vi "Receiver HMI Main.vi"() -> ()   [LabVIEW 2025]
uses:
  <vilib>/picture/picture.llb/Draw True-Color Pixmap.vi
  <vilib>/Instr/_visa.llb/VISA Configure Serial Port (Instr).vi
panel:
  out "Wire":bool
  out "Speaker":bool
  out "Motor":bool
  out "Light":bool
  out "Touch":bool
  out "Solenoid":bool
  out "Cancelled":bool
  out "Receive Buffer":string
  in  "Enable Wire":bool
  in  "Enable Speaker":bool
  in  "Enable Motor":bool
  in  "Enable Light":bool
  in  "Enable Touch":bool
  in  "Enable Solenoid":bool
  out "String":string
  out "2D Picture":picture
  out "Receiving Progress:":dbl(slide) scale=0.0..100.0
  # "RECEIVER"
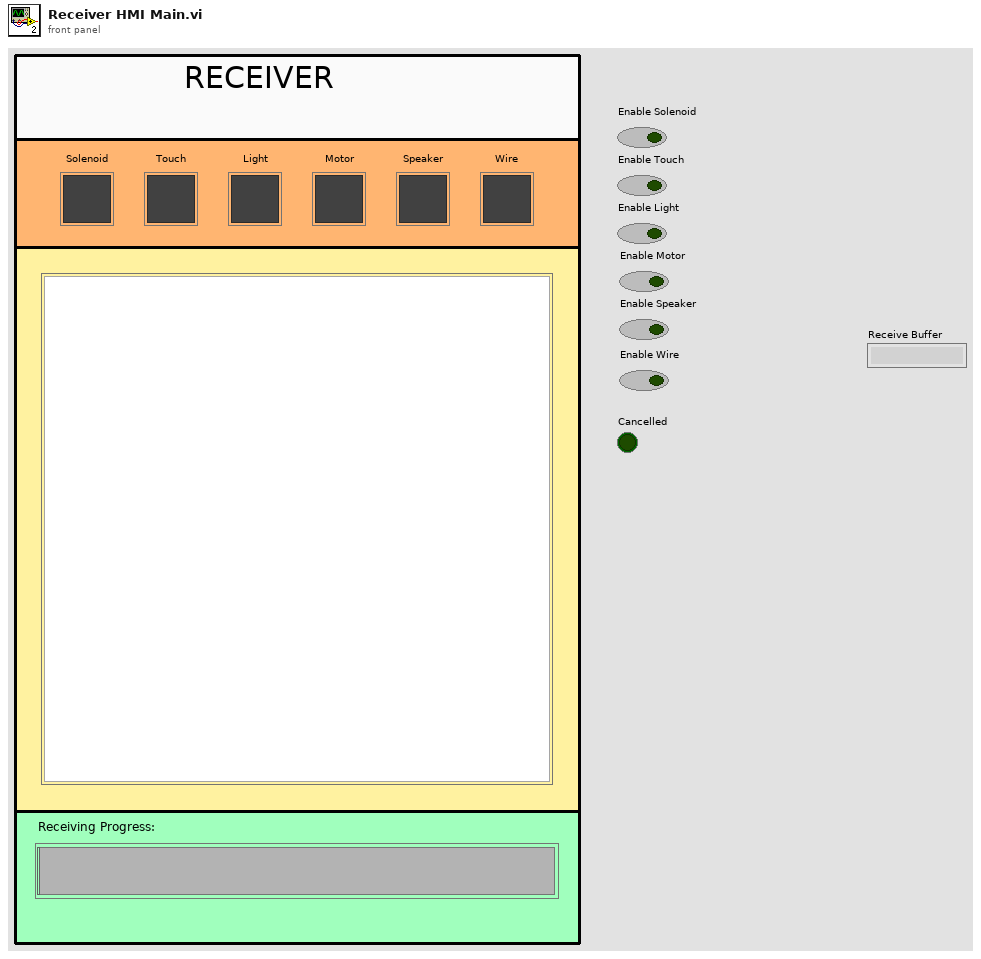
[diagram p1: front panel]
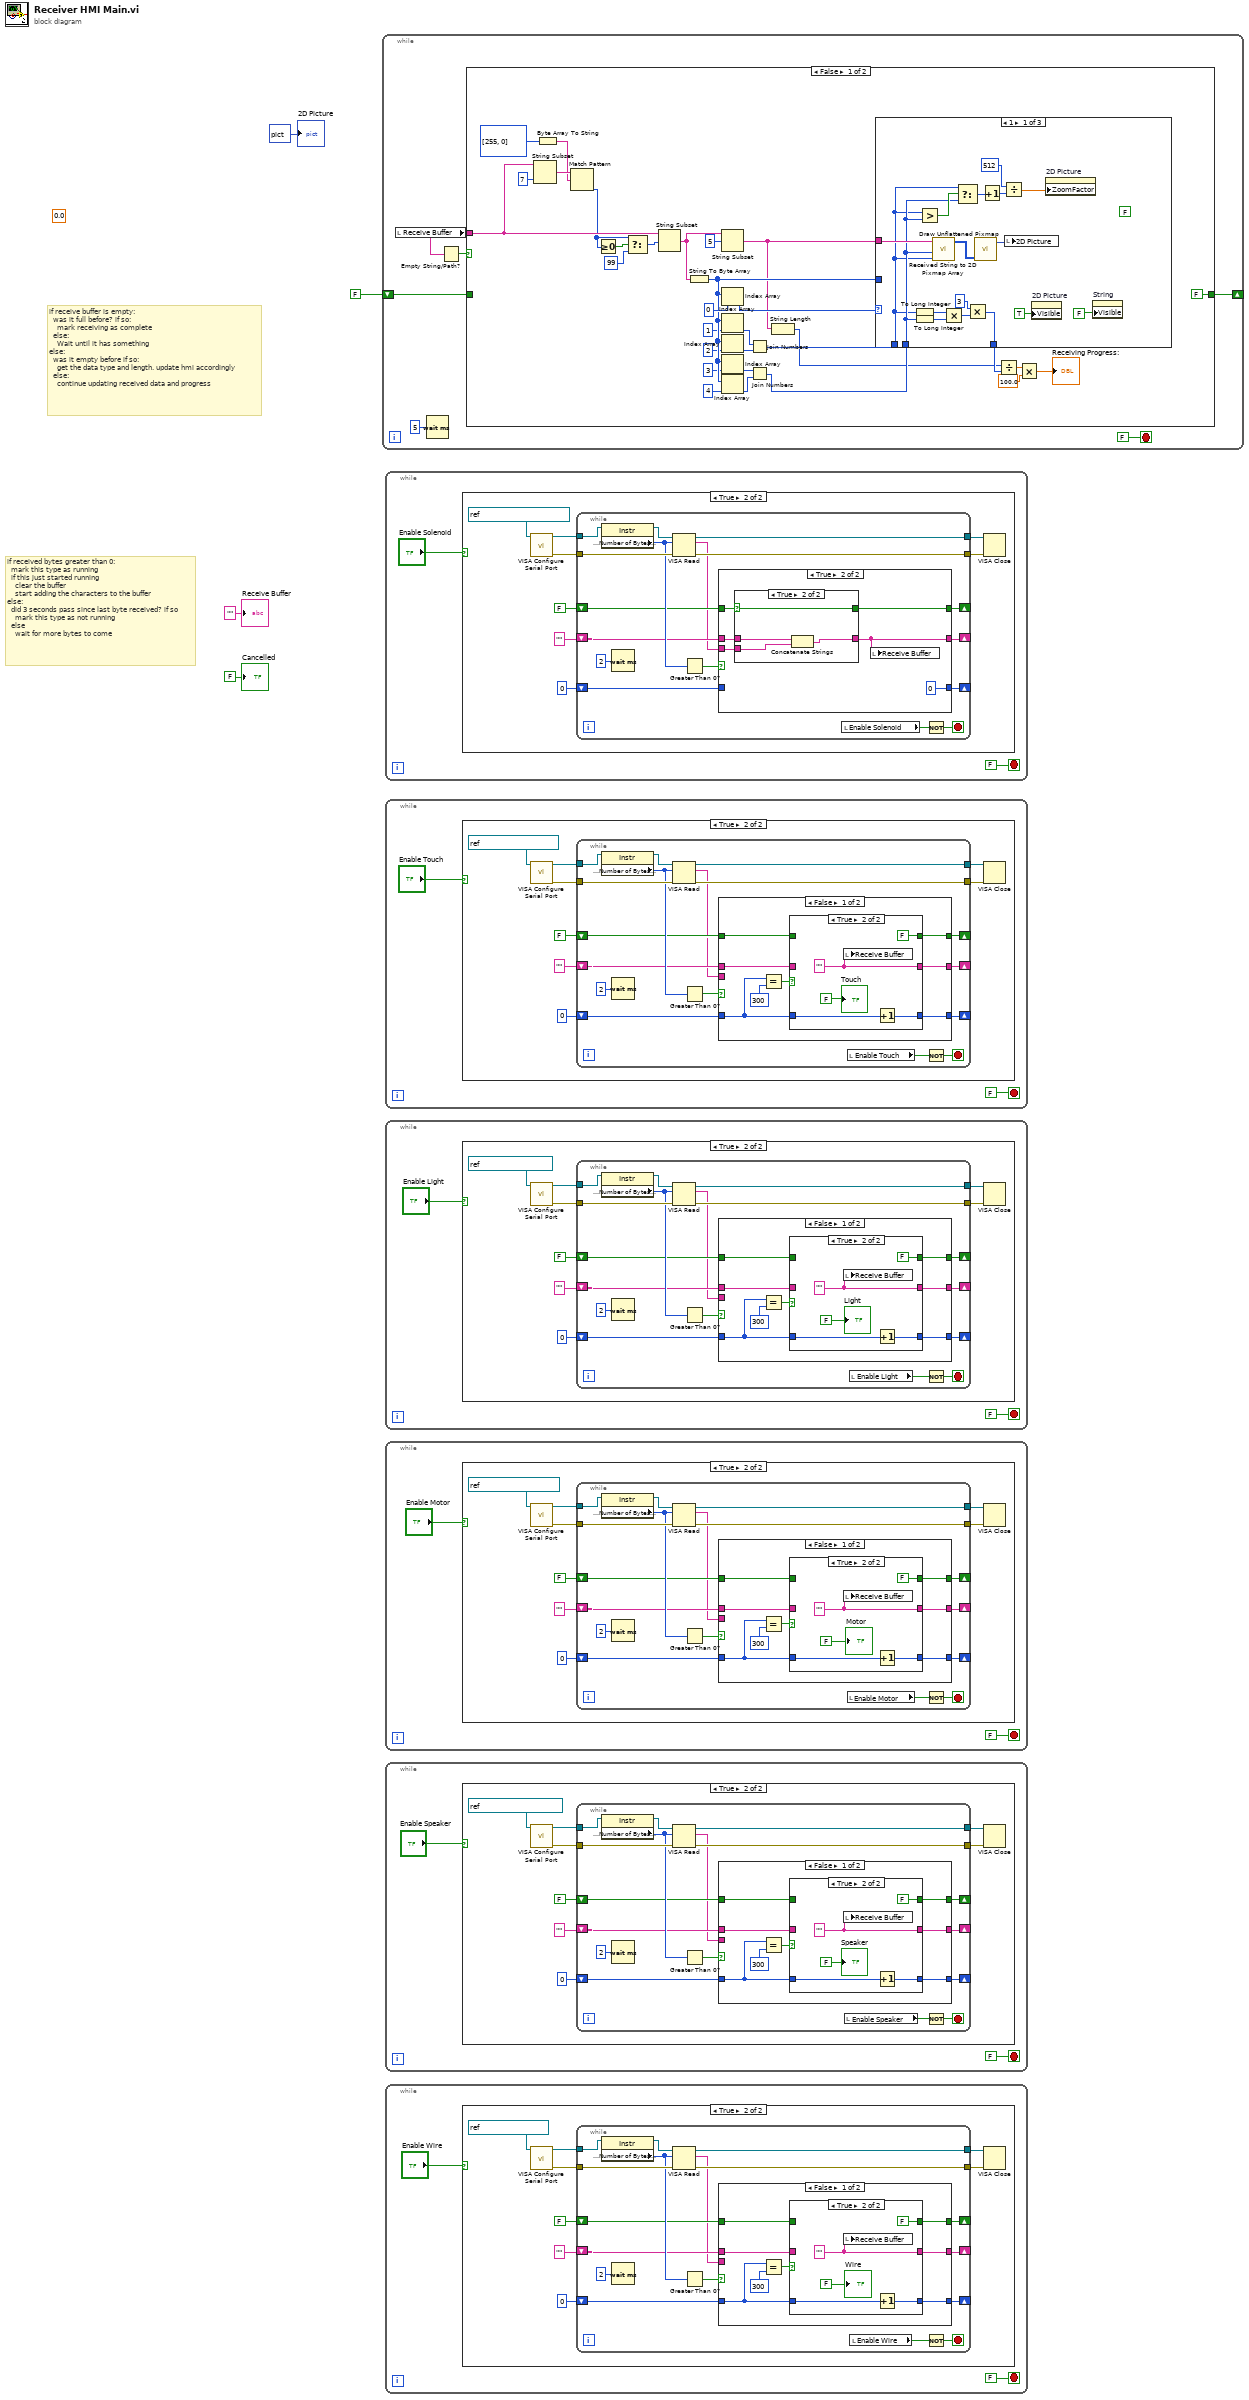
[diagram p0: block diagram]
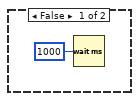
[diagram p2: hidden frame]
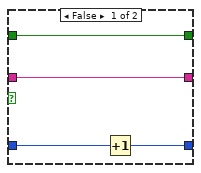
[diagram p3: hidden frame]
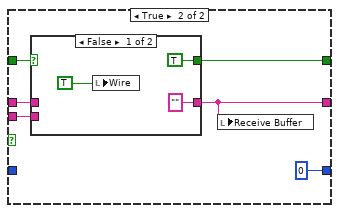
[diagram p4: hidden frame]
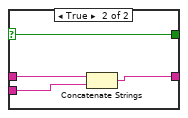
[diagram p5: hidden frame]
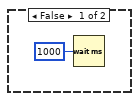
[diagram p6: hidden frame]
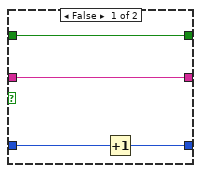
[diagram p7: hidden frame]
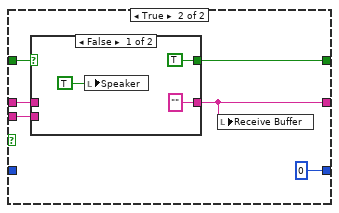
[diagram p8: hidden frame]
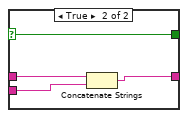
[diagram p9: hidden frame]
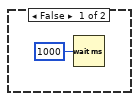
[diagram p10: hidden frame]
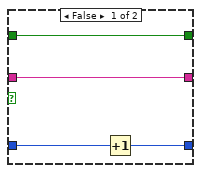
[diagram p11: hidden frame]
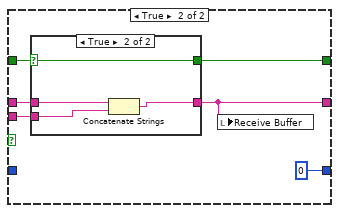
[diagram p12: hidden frame]
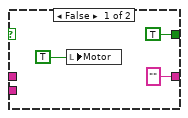
[diagram p13: hidden frame]
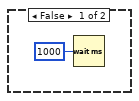
[diagram p14: hidden frame]
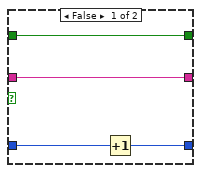
[diagram p15: hidden frame]
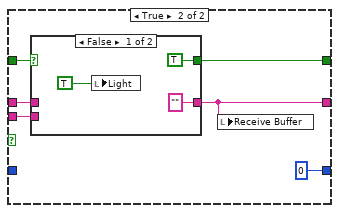
[diagram p16: hidden frame]
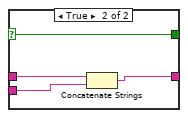
[diagram p17: hidden frame]
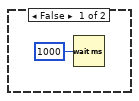
[diagram p18: hidden frame]
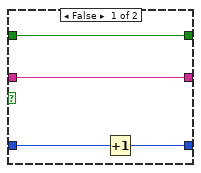
[diagram p19: hidden frame]
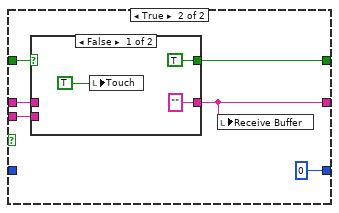
[diagram p20: hidden frame]
diagram:
  (unwired) 0.0 ("Receiving Progress:")
  # "if receive buffer is empty:\n  was it full before? if so:\n    mark receiving as complete\n  else:\n    Wait until it has something\nelse:\n  was it empty before if so:\n    get the data type and length. update hmi accordingly\n  else:\n    continue updating received data and progress"
  # "if received bytes greater than 0:\n  mark this type as running\n  if this just started running\n    clear the buffer\n    start adding the characters to the buffer\nelse:\n  did 3 seconds pass since last byte received? if so\n    mark this type as not running\n  else\n    wait for more bytes to come"
  n1 = while {
    shift-right: [w7] -> _
    shift-left: FALSE -> [w9]
    stop <- FALSE stop-if-true
    n2 = local read "Receive Buffer"() -> (w6:string)
    n3 = Wait (ms)(milliseconds to wait=u32 5) -> ()  [unwired: 1 out]
    n4 = Empty String/Path?(string/path=w6) -> (empty?=w10:bool)
    n5 = case shown="False" w10 {
      tunnel: w9 -> [_ w70]
      tunnel: [FALSE w69] -> w7
      tunnel: w6 -> [w19 _]
      frame False {
        n6 = String Subset(string=w19, length (rest)=7 ("length (rest)")) -> (substring=w21:string)  [unwired: 1 in]
        n7 = Byte Array To String(unsigned byte array=u8[] [255, 0]) -> (string=w20:string)
        n8 = Match Pattern(string=w21, regular expression=w20) -> (offset past match=w16:i32)  [unwired: 1 in, 3 out]
        n9 = Greater Or Equal To 0?(x=w16) -> (x >= 0?=w17:bool)
        n10 = Select(t=w16, s=w17, f=99) -> (s? t:f=w14:i32)
        n11 = String Subset(string=w19, offset (0)=w14) -> (substring=w18:string)  [unwired: 1 in]
        n12 = String To Byte Array(string=w18) -> (unsigned byte array=w32:u8[])
        n13 = String Subset(string=w18, offset (0)=5) -> (substring=w26:string)  [unwired: 1 in]
        n14 = Index Array(array=w32, index=0) -> (element=w40:u8)
        n15 = Index Array(array=w32, index=1) -> (element=w28:u8)
        n16 = Index Array(array=w32, index=2) -> (element=w27:u8)
        n17 = Index Array(array=w32, index=3) -> (element=w34:u8)
        n18 = Index Array(array=w32, index=4) -> (element=w33:u8)
        n19 = Join Numbers(hi=w28, lo=w27) -> ((hi.lo)=w25:u16)
        n20 = Join Numbers(hi=w34, lo=w33) -> ((hi.lo)=w24:u16)
        n21 = String Length(string=w26) -> (length=w12:i32)
        n22 = case shown="1" w40 {
          tunnel: w32 -> [_ _ _]
          tunnel: w26 -> [w56 _ w66]
          tunnel: w25 -> [w42 _ w64]
          tunnel: w24 -> [w44 _ w63]
          tunnel: [w52 u32 0 w62] -> w13
          frame 1 {
            (unwired) FALSE
            n23 = To Long Integer(number=w42) -> (32bit integer=w43:i32)
            n24 = To Long Integer(number=w44) -> (32bit integer=w45:i32)
            n25 = Greater?(x=w42, y=w44) -> (0:w50:bool)
            n26 = call "Received String to 2D Pixmap Array.vi"("Width"=w42, "Height"=w44, "Receive Buffer"=w56) -> ("Array"=w55:u32[][])  [unwired: 8 in]
            n27 = Multiply(x=w43, y=w45) -> (x*y=w54:i32)
            n28 = Select(t=w42, s=w50, f=w44) -> (s? t:f=w46:u16)
            n29 = Multiply(x=u16 3, y=w54) -> (x*y=w52:i32)
            n30 = call-poly <vilib>:"Draw Unflattened Pixmap.vi"("data (RGB format)"=w55) -> ("new picture"=w57:picture)  [unwired: 8 in]
            n31 = Increment(x=w46) -> (x+1=w47:u16)
            n32 = Divide(x=u16 512, y=w47) -> (x/y=w48:dbl)
            n33 = local write "2D Picture"(w57) -> ()
            n34 = property on="2D Picture" class="Pict"("Visible"=TRUE) -> ()  [unwired: 2 in, 2 out]
            n35 = property on="2D Picture" class="Pict"("ZoomFactor"=w48) -> ()  [unwired: 2 in, 2 out]
            n36 = property on="String" class="Str"("Visible"=FALSE) -> ()  [unwired: 2 in, 2 out]
          }
          frame Default {
            (unwired) FALSE
            n37 = local write "String"("INVALID DATA TYPE") -> ()
          }
          frame 0 {
            (unwired) TRUE
            n38 = property on="2D Picture" class="Pict"("Visible"=FALSE) -> ()  [unwired: 2 in, 2 out]
            n39 = property on="String" class="Str"("Visible"=TRUE) -> ()  [unwired: 2 in, 2 out]
            n40 = Join Numbers(hi=w64, lo=w63) -> ((hi.lo)=w62:u32)
            n41 = property on="String" class="Str"() -> ("Key Focus"=w67:bool)  [unwired: 2 in, 2 out]
            n42 = case shown="False" w67 {
              frame False {
                n43 = property on="String" class="Str"("Text.Scroll Position"=u32 65535) -> ()  [unwired: 2 in, 2 out]
              }
              frame True {
              }
            }
            "String" <- w66
          }
        }
        n44 = Divide(x=w12, y=w13) -> (x/y=w39:dbl)
        n45 = Multiply(x=w39, y=100.0) -> (x*y=→"Receiving Progress:":dbl)
      }
      frame True {
        n46 = case shown="True" w70 {
          selector: w70 -> [w71 _]
          tunnel: [w71 FALSE] -> w69
          frame False {
          }
          frame True {
            # "mark receiving as complete"
          }
        }
      }
    }
  }
  n47 = while {
    stop <- FALSE stop-if-true
    n48 = case shown="True" "Enable Solenoid" {
      frame False {
        n49 = Wait (ms)(milliseconds to wait=u32 1000) -> ()  [unwired: 1 out]
      }
      frame True {
        n50 = call-poly "VISA Configure Serial Port"("VISA resource name"=refnum<visa-resource-name> "SOLENOID_RECEIVER") -> ("VISA resource name out"=w82:refnum<visa-resource-name>, "error out"=w83:errorcluster)  [unwired: 13 in]
        n51 = while {
          tunnel: w83 -> [w100]
          tunnel: w82 -> [w98]
          shift-right: [w87] -> _
          shift-left: 0 -> [w86]
          shift-right: [w90] -> _
          shift-left: "" -> [w91]
          tunnel: [w96] -> w79
          tunnel: [w95] -> w78
          shift-right: [w88] -> _
          shift-left: FALSE -> [w92]
          stop <- w85 stop-if-true
          n52 = property class="Instr"(reference=w98) -> (reference out=w97:refnum<visa-resource-name>, "Serial Settings:Number of Bytes at Serial Port"=w93:u32)  [unwired: 1 in, 1 out]
          n53 = Wait (ms)(milliseconds to wait=u32 2) -> ()  [unwired: 1 out]
          n54 = VISA Read(VISA resource name=w97, byte count=w93, error in (no error)=w100) -> (VISA resource name out=w96:refnum<visa-resource-name>, read buffer=w89:string, error out=w95:errorcluster)  [unwired: 1 out]
          n55 = Greater Than 0?(x=w93) -> (x > 0?=w94:bool)
          n56 = case shown="True" w94 {
            tunnel: w92 -> [w101 w123]
            tunnel: w91 -> [w106 w122]
            tunnel: [w105 w118] -> w90
            tunnel: w89 -> [_ w121]
            tunnel: [w104 w120] -> w88
            tunnel: [w103 0] -> w87
            tunnel: w86 -> [w102 _]
            frame False {
              n57 = Equal?(x=w102, y=300) -> (x = y?=w107:bool)
              n58 = case shown="False" w107 {
                tunnel: w106 -> [w112 _]
                tunnel: [w112 w115] -> w105
                tunnel: [w111 FALSE] -> w104
                tunnel: [w109 w113] -> w103
                tunnel: w102 -> [w110 w114]
                tunnel: w101 -> [w111 _]
                frame False {
                  n59 = Increment(x=w110) -> (x+1=w109:i32)
                }
                frame True {
                  w115 = ""
                  n60 = local write "Receive Buffer"(w115) -> ()
                  n61 = Increment(x=w114) -> (x+1=w113:i32)
                  "Solenoid" <- FALSE ("Solenoid")
                }
              }
            }
            frame True {
              n62 = case shown="True" w123 {
                selector: w123 -> [_ w130]
                tunnel: w122 -> [_ w129]
                tunnel: ["" w128] -> w118
                tunnel: w121 -> [_ w127]
                tunnel: [TRUE w130] -> w120
                frame False {
                  n63 = local write "Solenoid"(TRUE ("Solenoid")) -> ()
                }
                frame True {
                  n64 = Concatenate Strings(w129, w127) -> (w128:string)
                }
              }
              n65 = local write "Receive Buffer"(w118) -> ()
            }
          }
          n66 = local read "Enable Solenoid"() -> (w84:bool)
          n67 = Not(x=w84) -> (.not. x?=w85:bool)
        }
        n68 = VISA Close(VISA resource name=w79, error in (no error)=w78) -> ()  [unwired: 1 out]
      }
    }
  }
  n69 = while {
    stop <- FALSE stop-if-true
    n70 = case shown="True" "Enable Touch" {
      frame False {
        n71 = Wait (ms)(milliseconds to wait=u32 1000) -> ()  [unwired: 1 out]
      }
      frame True {
        n72 = call-poly "VISA Configure Serial Port"("VISA resource name"=refnum<visa-resource-name> "TOUCH_RECEIVER") -> ("VISA resource name out"=w140:refnum<visa-resource-name>, "error out"=w141:errorcluster)  [unwired: 13 in]
        n73 = while {
          tunnel: w141 -> [w158]
          tunnel: w140 -> [w156]
          shift-right: [w145] -> _
          shift-left: 0 -> [w144]
          shift-right: [w148] -> _
          shift-left: "" -> [w149]
          tunnel: [w154] -> w137
          tunnel: [w153] -> w136
          shift-right: [w146] -> _
          shift-left: FALSE -> [w150]
          stop <- w143 stop-if-true
          n74 = property class="Instr"(reference=w156) -> (reference out=w155:refnum<visa-resource-name>, "Serial Settings:Number of Bytes at Serial Port"=w151:u32)  [unwired: 1 in, 1 out]
          n75 = Wait (ms)(milliseconds to wait=u32 2) -> ()  [unwired: 1 out]
          n76 = VISA Read(VISA resource name=w155, byte count=w151, error in (no error)=w158) -> (VISA resource name out=w154:refnum<visa-resource-name>, read buffer=w147:string, error out=w153:errorcluster)  [unwired: 1 out]
          n77 = Greater Than 0?(x=w151) -> (x > 0?=w152:bool)
          n78 = case shown="False" w152 {
            tunnel: w150 -> [w162 w181]
            tunnel: w149 -> [w166 w180]
            tunnel: [w165 w176] -> w148
            tunnel: w147 -> [_ w179]
            tunnel: [w164 w178] -> w146
            tunnel: [w163 0] -> w145
            tunnel: w144 -> [w160 _]
            frame False {
              n79 = Equal?(x=w160, y=300) -> (x = y?=w161:bool)
              n80 = case shown="True" w161 {
                tunnel: w166 -> [w170 _]
                tunnel: [w170 w174] -> w165
                tunnel: [w169 FALSE] -> w164
                tunnel: [w167 w171] -> w163
                tunnel: w160 -> [w168 w172]
                tunnel: w162 -> [w169 _]
                frame False {
                  n81 = Increment(x=w168) -> (x+1=w167:i32)
                }
                frame True {
                  w174 = ""
                  n82 = local write "Receive Buffer"(w174) -> ()
                  n83 = Increment(x=w172) -> (x+1=w171:i32)
                  "Touch" <- FALSE ("Solenoid")
                }
              }
            }
            frame True {
              n84 = case shown="False" w181 {
                selector: w181 -> [_ w188]
                tunnel: w180 -> [_ w187]
                tunnel: ["" w186] -> w176
                tunnel: w179 -> [_ w185]
                tunnel: [TRUE w188] -> w178
                frame False {
                  n85 = local write "Touch"(TRUE ("Solenoid")) -> ()
                }
                frame True {
                  n86 = Concatenate Strings(w187, w185) -> (w186:string)
                }
              }
              n87 = local write "Receive Buffer"(w176) -> ()
            }
          }
          n88 = local read "Enable Touch"() -> (w142:bool)
          n89 = Not(x=w142) -> (.not. x?=w143:bool)
        }
        n90 = VISA Close(VISA resource name=w137, error in (no error)=w136) -> ()  [unwired: 1 out]
      }
    }
  }
  n91 = while {
    stop <- FALSE stop-if-true
    n92 = case shown="True" "Enable Light" {
      frame False {
        n93 = Wait (ms)(milliseconds to wait=u32 1000) -> ()  [unwired: 1 out]
      }
      frame True {
        n94 = call-poly "VISA Configure Serial Port"("VISA resource name"=refnum<visa-resource-name> "LIGHT_RECEIVER") -> ("VISA resource name out"=w198:refnum<visa-resource-name>, "error out"=w199:errorcluster)  [unwired: 13 in]
        n95 = while {
          tunnel: w199 -> [w216]
          tunnel: w198 -> [w214]
          shift-right: [w203] -> _
          shift-left: 0 -> [w202]
          shift-right: [w206] -> _
          shift-left: "" -> [w207]
          tunnel: [w212] -> w195
          tunnel: [w211] -> w194
          shift-right: [w204] -> _
          shift-left: FALSE -> [w208]
          stop <- w201 stop-if-true
          n96 = property class="Instr"(reference=w214) -> (reference out=w213:refnum<visa-resource-name>, "Serial Settings:Number of Bytes at Serial Port"=w209:u32)  [unwired: 1 in, 1 out]
          n97 = Wait (ms)(milliseconds to wait=u32 2) -> ()  [unwired: 1 out]
          n98 = VISA Read(VISA resource name=w213, byte count=w209, error in (no error)=w216) -> (VISA resource name out=w212:refnum<visa-resource-name>, read buffer=w205:string, error out=w211:errorcluster)  [unwired: 1 out]
          n99 = Greater Than 0?(x=w209) -> (x > 0?=w210:bool)
          n100 = case shown="False" w210 {
            tunnel: w208 -> [w220 w239]
            tunnel: w207 -> [w224 w238]
            tunnel: [w223 w234] -> w206
            tunnel: w205 -> [_ w237]
            tunnel: [w222 w236] -> w204
            tunnel: [w221 0] -> w203
            tunnel: w202 -> [w218 _]
            frame False {
              n101 = Equal?(x=w218, y=300) -> (x = y?=w219:bool)
              n102 = case shown="True" w219 {
                tunnel: w224 -> [w228 _]
                tunnel: [w228 w232] -> w223
                tunnel: [w227 FALSE] -> w222
                tunnel: [w225 w230] -> w221
                tunnel: w218 -> [w226 w231]
                tunnel: w220 -> [w227 _]
                frame False {
                  n103 = Increment(x=w226) -> (x+1=w225:i32)
                }
                frame True {
                  w232 = ""
                  n104 = local write "Receive Buffer"(w232) -> ()
                  n105 = Increment(x=w231) -> (x+1=w230:i32)
                  "Light" <- FALSE ("Solenoid")
                }
              }
            }
            frame True {
              n106 = case shown="False" w239 {
                selector: w239 -> [_ w246]
                tunnel: w238 -> [_ w245]
                tunnel: ["" w244] -> w234
                tunnel: w237 -> [_ w243]
                tunnel: [TRUE w246] -> w236
                frame False {
                  n107 = local write "Light"(TRUE ("Solenoid")) -> ()
                }
                frame True {
                  n108 = Concatenate Strings(w245, w243) -> (w244:string)
                }
              }
              n109 = local write "Receive Buffer"(w234) -> ()
            }
          }
          n110 = local read "Enable Light"() -> (w200:bool)
          n111 = Not(x=w200) -> (.not. x?=w201:bool)
        }
        n112 = VISA Close(VISA resource name=w195, error in (no error)=w194) -> ()  [unwired: 1 out]
      }
    }
  }
  n113 = while {
    stop <- FALSE stop-if-true
    n114 = case shown="True" "Enable Motor" {
      frame False {
        n115 = Wait (ms)(milliseconds to wait=u32 1000) -> ()  [unwired: 1 out]
      }
      frame True {
        n116 = call-poly "VISA Configure Serial Port"("VISA resource name"=refnum<visa-resource-name> "MOTOR_RECEIVER") -> ("VISA resource name out"=w256:refnum<visa-resource-name>, "error out"=w257:errorcluster)  [unwired: 13 in]
        n117 = while {
          tunnel: w257 -> [w274]
          tunnel: w256 -> [w272]
          shift-right: [w261] -> _
          shift-left: 0 -> [w260]
          shift-right: [w264] -> _
          shift-left: "" -> [w265]
          tunnel: [w270] -> w253
          tunnel: [w269] -> w252
          shift-right: [w262] -> _
          shift-left: FALSE -> [w266]
          stop <- w259 stop-if-true
          n118 = property class="Instr"(reference=w272) -> (reference out=w271:refnum<visa-resource-name>, "Serial Settings:Number of Bytes at Serial Port"=w267:u32)  [unwired: 1 in, 1 out]
          n119 = Wait (ms)(milliseconds to wait=u32 2) -> ()  [unwired: 1 out]
          n120 = VISA Read(VISA resource name=w271, byte count=w267, error in (no error)=w274) -> (VISA resource name out=w270:refnum<visa-resource-name>, read buffer=w263:string, error out=w269:errorcluster)  [unwired: 1 out]
          n121 = Greater Than 0?(x=w267) -> (x > 0?=w268:bool)
          n122 = case shown="False" w268 {
            tunnel: w266 -> [w278 w297]
            tunnel: w265 -> [w282 w296]
            tunnel: [w281 w292] -> w264
            tunnel: w263 -> [_ w295]
            tunnel: [w280 w294] -> w262
            tunnel: [w279 0] -> w261
            tunnel: w260 -> [w276 _]
            frame False {
              n123 = Equal?(x=w276, y=300) -> (x = y?=w277:bool)
              n124 = case shown="True" w277 {
                tunnel: w282 -> [w286 _]
                tunnel: [w286 w290] -> w281
                tunnel: [w285 FALSE] -> w280
                tunnel: [w283 w288] -> w279
                tunnel: w276 -> [w284 w289]
                tunnel: w278 -> [w285 _]
                frame False {
                  n125 = Increment(x=w284) -> (x+1=w283:i32)
                }
                frame True {
                  w290 = ""
                  n126 = local write "Receive Buffer"(w290) -> ()
                  n127 = Increment(x=w289) -> (x+1=w288:i32)
                  "Motor" <- FALSE ("Solenoid")
                }
              }
            }
            frame True {
              n128 = case shown="True" w297 {
                selector: w297 -> [_ w304]
                tunnel: w296 -> [_ w303]
                tunnel: ["" w302] -> w292
                tunnel: w295 -> [_ w301]
                tunnel: [TRUE w304] -> w294
                frame False {
                  n129 = local write "Motor"(TRUE ("Solenoid")) -> ()
                }
                frame True {
                  n130 = Concatenate Strings(w303, w301) -> (w302:string)
                }
              }
              n131 = local write "Receive Buffer"(w292) -> ()
            }
          }
          n132 = local read "Enable Motor"() -> (w258:bool)
          n133 = Not(x=w258) -> (.not. x?=w259:bool)
        }
        n134 = VISA Close(VISA resource name=w253, error in (no error)=w252) -> ()  [unwired: 1 out]
      }
    }
  }
  n135 = while {
    stop <- FALSE stop-if-true
    n136 = case shown="True" "Enable Speaker" {
      frame False {
        n137 = Wait (ms)(milliseconds to wait=u32 1000) -> ()  [unwired: 1 out]
      }
      frame True {
        n138 = call-poly "VISA Configure Serial Port"("VISA resource name"=refnum<visa-resource-name> "SPEAKER_RECEIVER") -> ("VISA resource name out"=w314:refnum<visa-resource-name>, "error out"=w315:errorcluster)  [unwired: 13 in]
        n139 = while {
          tunnel: w315 -> [w332]
          tunnel: w314 -> [w330]
          shift-right: [w319] -> _
          shift-left: 0 -> [w318]
          shift-right: [w322] -> _
          shift-left: "" -> [w323]
          tunnel: [w328] -> w311
          tunnel: [w327] -> w310
          shift-right: [w320] -> _
          shift-left: FALSE -> [w324]
          stop <- w317 stop-if-true
          n140 = property class="Instr"(reference=w330) -> (reference out=w329:refnum<visa-resource-name>, "Serial Settings:Number of Bytes at Serial Port"=w325:u32)  [unwired: 1 in, 1 out]
          n141 = Wait (ms)(milliseconds to wait=u32 2) -> ()  [unwired: 1 out]
          n142 = VISA Read(VISA resource name=w329, byte count=w325, error in (no error)=w332) -> (VISA resource name out=w328:refnum<visa-resource-name>, read buffer=w321:string, error out=w327:errorcluster)  [unwired: 1 out]
          n143 = Greater Than 0?(x=w325) -> (x > 0?=w326:bool)
          n144 = case shown="False" w326 {
            tunnel: w324 -> [w336 w355]
            tunnel: w323 -> [w340 w354]
            tunnel: [w339 w350] -> w322
            tunnel: w321 -> [_ w353]
            tunnel: [w338 w352] -> w320
            tunnel: [w337 0] -> w319
            tunnel: w318 -> [w334 _]
            frame False {
              n145 = Equal?(x=w334, y=300) -> (x = y?=w335:bool)
              n146 = case shown="True" w335 {
                tunnel: w340 -> [w344 _]
                tunnel: [w344 w348] -> w339
                tunnel: [w343 FALSE] -> w338
                tunnel: [w341 w346] -> w337
                tunnel: w334 -> [w342 w347]
                tunnel: w336 -> [w343 _]
                frame False {
                  n147 = Increment(x=w342) -> (x+1=w341:i32)
                }
                frame True {
                  w348 = ""
                  n148 = local write "Receive Buffer"(w348) -> ()
                  n149 = Increment(x=w347) -> (x+1=w346:i32)
                  "Speaker" <- FALSE ("Solenoid")
                }
              }
            }
            frame True {
              n150 = case shown="False" w355 {
                selector: w355 -> [_ w362]
                tunnel: w354 -> [_ w361]
                tunnel: ["" w360] -> w350
                tunnel: w353 -> [_ w359]
                tunnel: [TRUE w362] -> w352
                frame False {
                  n151 = local write "Speaker"(TRUE ("Solenoid")) -> ()
                }
                frame True {
                  n152 = Concatenate Strings(w361, w359) -> (w360:string)
                }
              }
              n153 = local write "Receive Buffer"(w350) -> ()
            }
          }
          n154 = local read "Enable Speaker"() -> (w316:bool)
          n155 = Not(x=w316) -> (.not. x?=w317:bool)
        }
        n156 = VISA Close(VISA resource name=w311, error in (no error)=w310) -> ()  [unwired: 1 out]
      }
    }
  }
  n157 = while {
    stop <- FALSE stop-if-true
    n158 = case shown="True" "Enable Wire" {
      frame False {
        n159 = Wait (ms)(milliseconds to wait=u32 1000) -> ()  [unwired: 1 out]
      }
      frame True {
        n160 = call-poly "VISA Configure Serial Port"("VISA resource name"=refnum<visa-resource-name> "WIRE_RECEIVER") -> ("VISA resource name out"=w372:refnum<visa-resource-name>, "error out"=w373:errorcluster)  [unwired: 13 in]
        n161 = while {
          tunnel: w373 -> [w390]
          tunnel: w372 -> [w388]
          shift-right: [w377] -> _
          shift-left: 0 -> [w376]
          shift-right: [w380] -> _
          shift-left: "" -> [w381]
          tunnel: [w386] -> w369
          tunnel: [w385] -> w368
          shift-right: [w378] -> _
          shift-left: FALSE -> [w382]
          stop <- w375 stop-if-true
          n162 = property class="Instr"(reference=w388) -> (reference out=w387:refnum<visa-resource-name>, "Serial Settings:Number of Bytes at Serial Port"=w383:u32)  [unwired: 1 in, 1 out]
          n163 = Wait (ms)(milliseconds to wait=u32 2) -> ()  [unwired: 1 out]
          n164 = VISA Read(VISA resource name=w387, byte count=w383, error in (no error)=w390) -> (VISA resource name out=w386:refnum<visa-resource-name>, read buffer=w379:string, error out=w385:errorcluster)  [unwired: 1 out]
          n165 = Greater Than 0?(x=w383) -> (x > 0?=w384:bool)
          n166 = case shown="False" w384 {
            tunnel: w382 -> [w394 w413]
            tunnel: w381 -> [w398 w412]
            tunnel: [w397 w408] -> w380
            tunnel: w379 -> [_ w411]
            tunnel: [w396 w410] -> w378
            tunnel: [w395 0] -> w377
            tunnel: w376 -> [w392 _]
            frame False {
              n167 = Equal?(x=w392, y=300) -> (x = y?=w393:bool)
              n168 = case shown="True" w393 {
                tunnel: w398 -> [w402 _]
                tunnel: [w402 w406] -> w397
                tunnel: [w401 FALSE] -> w396
                tunnel: [w399 w404] -> w395
                tunnel: w392 -> [w400 w405]
                tunnel: w394 -> [w401 _]
                frame False {
                  n169 = Increment(x=w400) -> (x+1=w399:i32)
                }
                frame True {
                  w406 = ""
                  n170 = local write "Receive Buffer"(w406) -> ()
                  n171 = Increment(x=w405) -> (x+1=w404:i32)
                  "Wire" <- FALSE ("Solenoid")
                }
              }
            }
            frame True {
              n172 = case shown="False" w413 {
                selector: w413 -> [_ w420]
                tunnel: w412 -> [_ w419]
                tunnel: ["" w418] -> w408
                tunnel: w411 -> [_ w417]
                tunnel: [TRUE w420] -> w410
                frame False {
                  n173 = local write "Wire"(TRUE ("Solenoid")) -> ()
                }
                frame True {
                  n174 = Concatenate Strings(w419, w417) -> (w418:string)
                }
              }
              n175 = local write "Receive Buffer"(w408) -> ()
            }
          }
          n176 = local read "Enable Wire"() -> (w374:bool)
          n177 = Not(x=w374) -> (.not. x?=w375:bool)
        }
        n178 = VISA Close(VISA resource name=w369, error in (no error)=w368) -> ()  [unwired: 1 out]
      }
    }
  }
  "Cancelled" <- FALSE ("Cancelled")
  "Receive Buffer" <- "" ("read buffer")
  "2D Picture" <- picture data[5B] ("2D Picture")
